vi "File Name Generator1.vi"(1 "FileName":string="data") -> (0 "File Name":string)   [LabVIEW 2018]
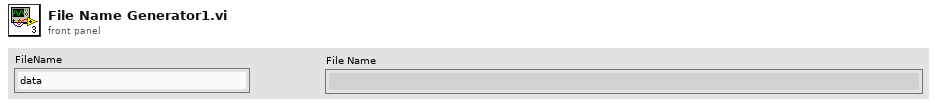
[diagram p1: front panel]
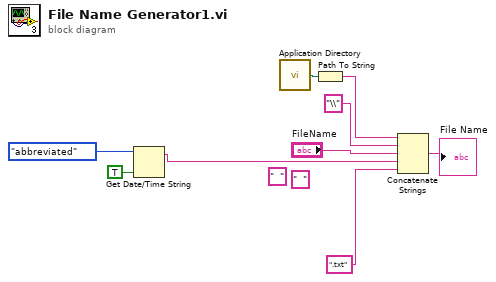
[diagram p0: block diagram]
diagram:
  (unwired) "  " ("string")
  (unwired) "  " ("string")
  n1 = Get Date/Time String(date format (0)=enum16{"short", "long", "abbreviated"}."abbreviated", want seconds? (F)=TRUE) -> (date string=w2:string)  [unwired: 1 in, 1 out]
  n2 = call <vilib>:"Application Directory.vi"() -> ("Application Directory"=w7:path)
  n3 = Path To String(path=w7) -> (string=w8:string)
  n4 = Concatenate Strings(w8, "\\" ("string"), "FileName", w2, ".txt" ("string")) -> (→"File Name":string)
